vi "Testbench.vi"() -> ()   [LabVIEW 2021]
uses:
  Source/FPGA/Neopixel - FPGA.lvclass
panel:
  out "Waveform Chart":i16(graph)
  in  "stop":bool
  in  "Enqueue":bool
  in  "Data":u8[](array[numeric])
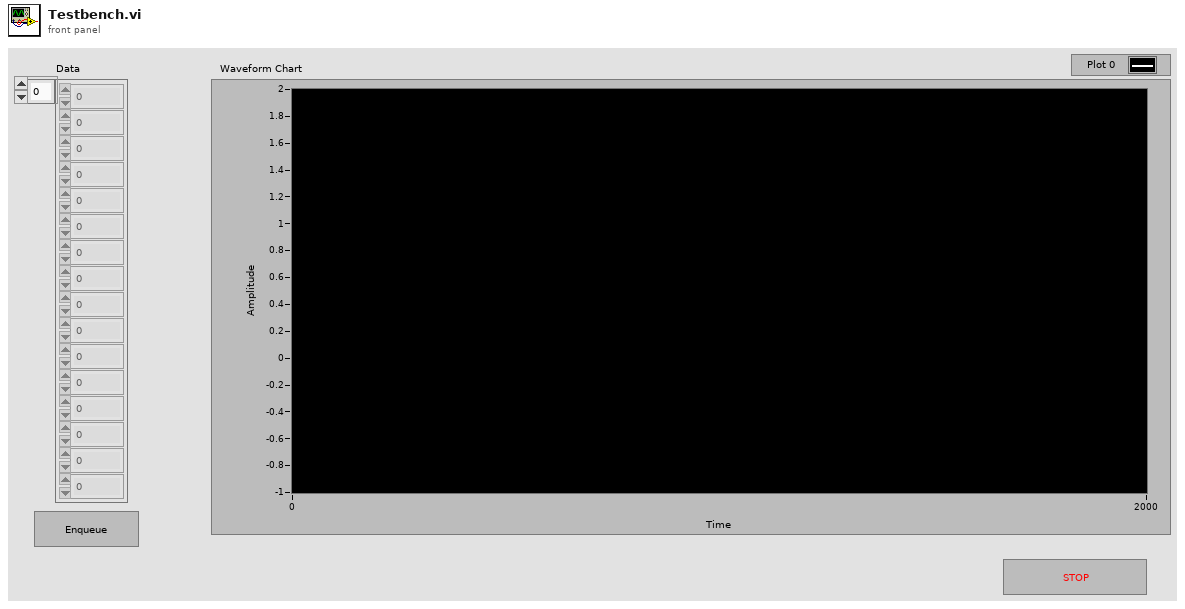
[diagram p1: front panel]
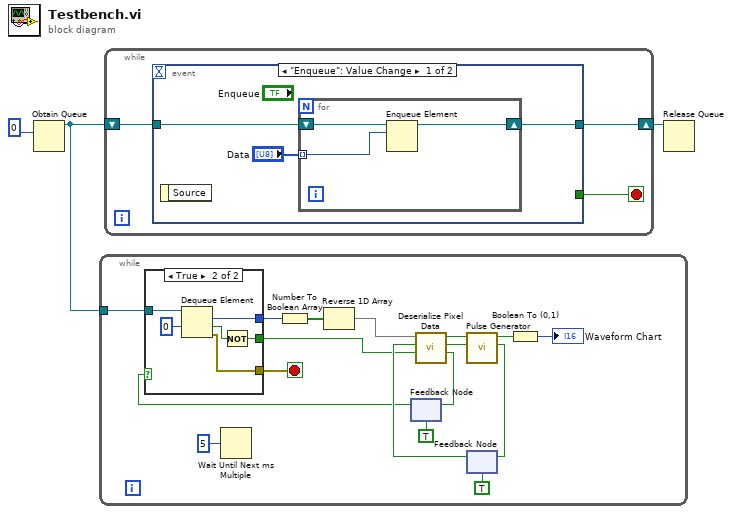
[diagram p0: block diagram]
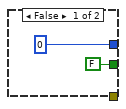
[diagram p2: hidden frame]
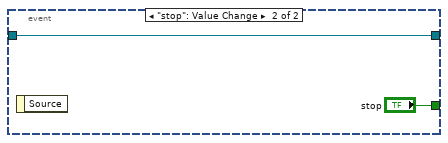
[diagram p3: hidden frame]
diagram:
  n1 = Obtain Queue(element data type=u8 0 ("Numeric")) -> (queue out=w1:refnum<queue>)  [unwired: 4 in, 2 out]
  n2 = while {
    tunnel: w1 -> [w14]
    stop <- w11 stop-if-true
    n3 = Wait Until Next ms Multiple(millisecond multiple=u32 5) -> ()  [unwired: 1 out]
    n4 = feedback #1(TRUE ("Value Reached")) -> (w9:bool)
    n5 = case shown="True" w9 {
      tunnel: w14 -> [_ w28]
      tunnel: [_ w27] -> w11
      tunnel: [u8 0 ("Numeric") w26] -> w8
      tunnel: [FALSE w23] -> w7
      frame False {
      }
      frame True {
        n6 = Dequeue Element(queue=w28, timeout in ms (-1)=0) -> (element=w26:u8, timed out?=w24:bool, error out=w27:errorcluster)  [unwired: 1 in, 1 out]
        n7 = Not(x=w24) -> (.not. x?=w23:bool)
      }
    }
    n8 = Number To Boolean Array(number=w8) -> (Boolean array=w20:bool[])
    n9 = Reverse 1D Array(array=w20) -> (reversed array=w19:bool[])
    n10 = feedback #2(TRUE ("Value Reached")) -> (w15:bool)
    n11 = call "Deserialize Pixel Data.vi"("Input Valid"=w7, "Ready For Output"=w15, "Pixel Data"=w19) -> ("Ready For Input"=w4:bool, "Output Valid"=w5:bool, "Deserialized Data"=w6:bool)  [unwired: 6 in]
    n12 = feedback-in #1(w4) -> ()
    n13 = call "Pulse Generator.vi"("Input Valid"=w5, "Data"=w6) -> ("Ready For Input"=w16:bool, "Pulse Output"=w13:bool)  [unwired: 8 in]
    n14 = feedback-in #2(w16) -> ()
    n15 = Boolean To (0,1)(Boolean=w13) -> (0, 1=→"Waveform Chart":i16)
  }
  n16 = while {
    shift-right: [w30] -> w2
    shift-left: w1 -> [w31]
    stop <- w29 stop-if-true
    n17 = event shown="[0] \"Enqueue\": Value Change" {
      selector: _ -> [_ _]
      dyn-events: _ -> [_ _]
      timeout: _ -> [_ _]
      tunnel: w31 -> [w34 w38]
      tunnel: [w33 w38] -> w30
      tunnel: [_ "stop"] -> w29
      event "Enqueue": Value Change {
        n18 = event-data() -> ()  [unwired: 1 in, 1 out]
        n19 = for {
          shift-right: [w36] -> w33
          shift-left: w34 -> [w37]
          tunnel: "Data" -> [w35] mode=indexing
          n20 = Enqueue Element(queue=w37, element=w35) -> (queue out=w36:refnum<queue>)  [unwired: 2 in, 2 out]
        }
      }
      event "stop": Value Change {
        n21 = event-data() -> ()  [unwired: 1 in, 1 out]
      }
    }
  }
  n22 = Release Queue(queue=w2) -> ()  [unwired: 2 in, 3 out]
